vi "ClusterEscala.vi"() -> ()   [LabVIEW 2020]
panel:
  out "Resultado":T1 {"Gauge" scale=0.0..100.0; "Tank" scale=0.0..15.0; "Thermometer" scale=0.0..100.0}
  in  "Entradas":T2
  # "Diego Jáuregui Ontiveros\nCarlos Uriel Casas Casas\nAlejandro López González"
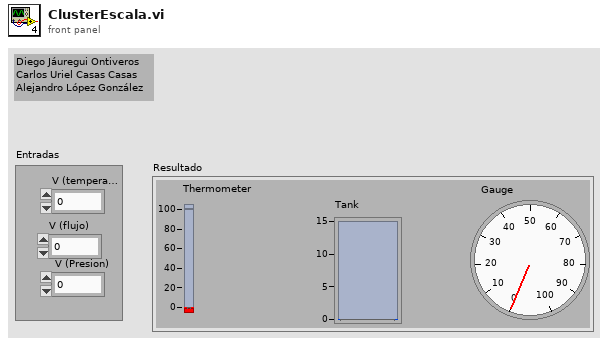
[diagram p1: front panel]
types:
  T1 = cluster{"Thermometer":dbl, "Tank":dbl, "Gauge":dbl}
  T2 = cluster{"V (temperatura)":dbl, "V (flujo) ":dbl, " V (Presion)":dbl}
  T3 = cluster{"°C/V":i32, "(l/seg)/V":i32, "(N/m^2)/V":i32}
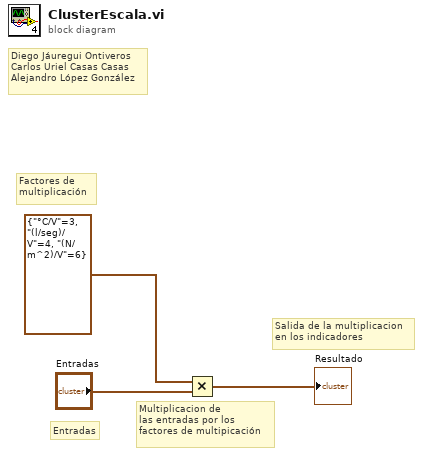
[diagram p0: block diagram]
diagram:
  # "Diego Jáuregui Ontiveros\nCarlos Uriel Casas Casas\nAlejandro López González"
  # "Salida de la multiplicacion\nen los indicadores"
  # "Multiplicacion de \nlas entradas por los\nfactores de multipicación"
  # "Entradas"
  # "Factores de \nmultiplicación"
  n1 = Multiply(x=T3 {"°C/V"=3, "(l/seg)/V"=4, "(N/m^2)/V"=6} ("Cluster"), y="Entradas") -> (x*y=→"Resultado":cluster{dbl, dbl, dbl})
